vi "Get DAQ Status.vi"(8 "error in (no error)":errorcluster, 11 "DAQ Manager in":refnum<class "DAQ Manager.lvclass">=refnum) -> (0 "error out":errorcluster, 1 "TCP Port Number":u32, 2 "Run Number":u32, 3 "DAQ Manager out":refnum<class "DAQ Manager.lvclass">, 4 "Data storage path":string, 5 "Run Active?":bool)   [LabVIEW 2020, in "CIRCUS_uServices.lvlib" / "DAQ Manager.lvlib" / "DAQ Manager.lvclass"]
uses:
  DAQ Manager.lvclass
  DAQ Manager.lvclass/DAQ Manager.ctl
  TALOS/TALOS_PPL.lvlibp/Interfaces/DAQ Control/DAQ Control.lvclass
  TALOS/TALOS_PPL.lvlibp
  C:/Users/marco/Documents/GitHub_Lab/CIRCUS/TALOS/TALOS_PPL.lvlibp/Father of all uServices/Father of all uServices/Father of all uServices.lvclass
  C:/Users/marco/Documents/GitHub_Lab/CIRCUS/TALOS/TALOS_PPL.lvlibp/Ancestor/Ancestor/Ancestor.lvclass
  C:/Users/marco/Documents/GitHub_Lab/CIRCUS/TALOS/Actor Framework.lvlibp/1abvi3w/vi.lib/ActorFramework/Actor/Actor.lvclass
  C:/Users/marco/Documents/GitHub_Lab/CIRCUS/CIRCUS uServices et al/DAQ Manager/DAQ Manager.lvclass
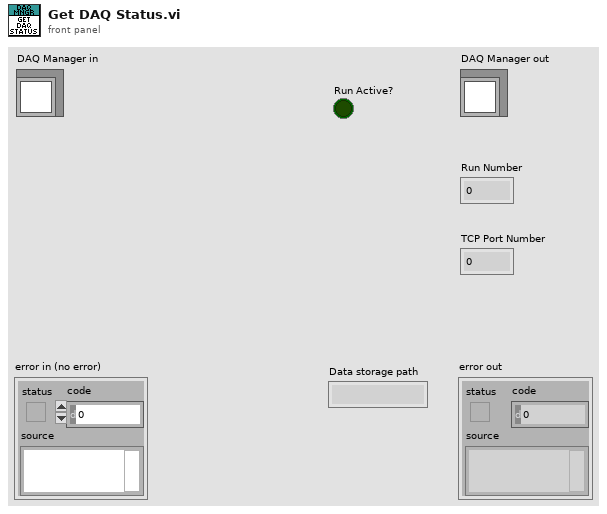
[diagram p1: front panel]
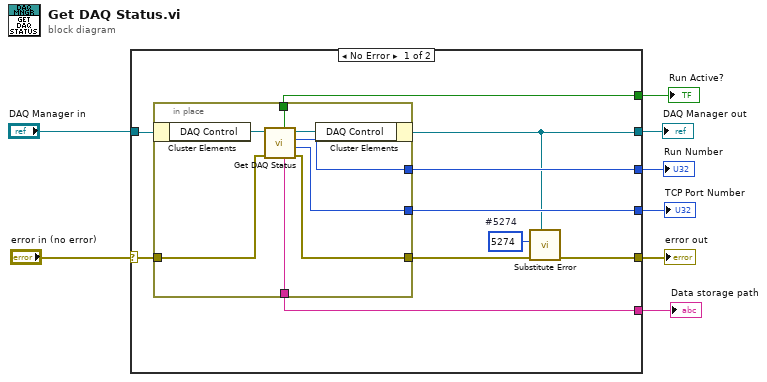
[diagram p0: block diagram]
diagram:
  n1 = case shown="No Error" "error in (no error)" {
    selector: "error in (no error)" -> [w17 w28]
    tunnel: [w11 w28] -> w7
    tunnel: [w10 w27] -> w5
    tunnel: "DAQ Manager in" -> [w18 w27]
    tunnel: [w16 _] -> w4
    tunnel: [w15 _] -> w3
    tunnel: [w14 _] -> w2
    tunnel: [w13 _] -> w1
    frame No Error {
      w9 = 5274  # #5274
      n2 = in-place {
        in-place-border: w17 -> [w23]
        in-place-border: [w22] -> w12
        in-place-border: [w20] -> w16
        in-place-border: [w24] -> w15
        in-place-border: [w21] -> w14
        in-place-border: [w19] -> w13
        n3 = in-place-cluster #1(w18) -> ("DAQ Control"=w26:refnum<class "DAQ Control.lvclass">)
        n4 = call-dynamic "Get DAQ Status.vi"("error in (no error)"=w23, "DAQ Control in"=w26) -> ("error out"=w22:errorcluster, "TCP Port Number"=w21:u32, "Run Number"=w20:u32, "DAQ Control out"=w25:refnum<class "DAQ Control.lvclass">, "Data storage path"=w19:string, "Run Active?"=w24:bool)  [unwired: 4 in]
        n5 = in-place-cluster #1("DAQ Control"=w25) -> (w10:refnum<class "DAQ Manager.lvclass">)
      }
      n6 = call "Substitute Error.vi"("LabVIEW Object"=w10, "error in (no error)"=w12, "Error Code"=w9) -> ("error out"=w11:errorcluster)  [unwired: 8 in]
    }
    frame Error {
    }
  }
  "error out" <- w7
  "DAQ Manager out" <- w5
  "Run Number" <- w4
  "Run Active?" <- w3
  "TCP Port Number" <- w2
  "Data storage path" <- w1
